vi "Matrix left divisionMV_general_direct.vi"(2 "A":dbl[](array[numeric]), 4 "B":dbl[][](array[numeric])) -> (0 "error":i32, 1 "B\\A":dbl[](array[numeric]))   [LabVIEW 2010, in "NI_Gmath.lvlib"]
doc: "Left division operator. B\\A solves the equation B*X=A. When used with two polynomials, \\ is overloaded to produce a transfer function whose numerator is the right-hand operand. When used with two dynamic systems, a new system is created whose state matrix is the appended states of the two systems and whose output matrix is that of the \"numerator\" system. (For systems in transfer- function format, the new system is obtained by multiplying the \"numerator\" system by the reciprocal of the \"denominator\" system.) For matrix division, there are no specific conditions on the dimensions of A and B but the condition of B affects the accuracy of the matrix quotient obtained. An error message appears if B is singular. If B is square and nonsingular, B\\A returns a matrix X with the same dimensions as A. An LU (Gaussian) decomposition, rather than a direct inverse, is used. If the condition estimate of B is less than the machine epsilon, a warning message appears. If B is non-square, X is the least-squares solution to B*X=A and has row dimension equal to the number of columns of B and column dimension equal to the number of columns of A. This operation uses a QR decomposition to implicitly compute the rank of B; the solution X will have no more nonzero components in each column than this rank value."
uses:
  NI_Gmath.lvlib
  Real PseudoInverse Matrix.vi
  A x Vector.vi
  NI_AALBase.lvlib
  NI_AALPro.lvlib
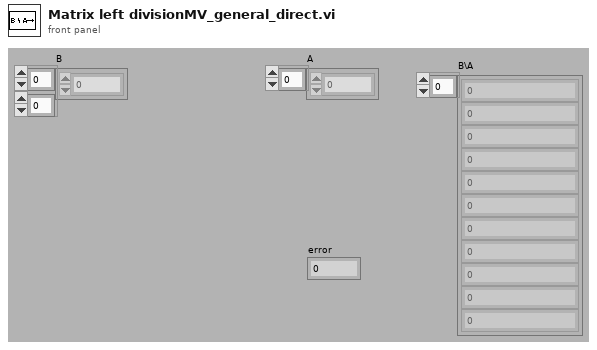
[diagram p1: front panel]
types:
  T1 = typedef "NI_Matrix.lvlib/RealMatrix.ctl" = dbl[][]
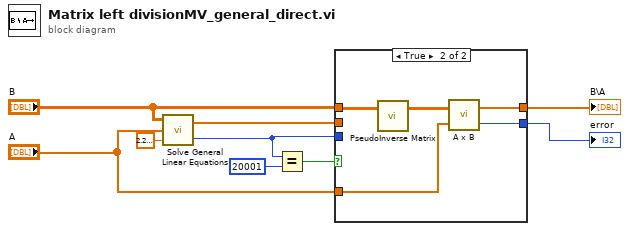
[diagram p0: block diagram]
diagram:
  n1 = call "Solve General Linear Equations.vi"("relative tolerance"=2.220446049250313e-16, "Known Vector"="A", "Input Matrix"="B") -> ("error"=w2:i32, "Solution Vector"=w3:dbl[])
  n2 = Equal?(x=w2, y=20001) -> (x = y?=w4:bool)
  n3 = case shown="True" w4 {
    tunnel: "B" -> [_ w16]
    tunnel: [w10 w12] -> w6
    tunnel: "A" -> [_ w14]
    tunnel: [w11 w13] -> w9
    tunnel: w2 -> [w11 _]
    tunnel: w3 -> [w10 _]
    frame False {
    }
    frame True {
      n4 = call-poly "PseudoInverse Matrix.vi"("Input Matrix"=w16) -> ("PseudoInverse Matrix"=w15:T1)  [unwired: 1 in, 1 out]
      n5 = call-poly "A x B.vi"("Vector"=w14, "A"=w15) -> ("error"=w13:i32, "A x Vector"=w12:dbl[])
    }
  }
  "B\\A" <- w6
  "error" <- w9
